vi "Extractor de bloobs.vi"() -> ()   [LabVIEW 2012]
doc: "Use this template to build a producer/consumer design pattern. Use this template when you need to execute a process, such as data analysis, when a data source, such as a triggered acquisition, produces data at an uneven rate and you need to execute the process when the data becomes available."
uses:
  <vilib>/vision/Image Controls.llb/IMAQ Image.ctl
  <vilib>/vision/NI_Vision_Development_Module.lvlib
panel:
  in  "Forma":i32=9
  in  "Tamaño":i32=50
  in  "Aguacate":bool
  out "Guardado":bool
  in  "Guardar":bool
  out "Image 2":T1(plugin-control)
  out "Cuadro":i32[](array[numeric])
  out "Image":T1(plugin-control)
  in  "Image\n  Path":path
  in  "stop":bool
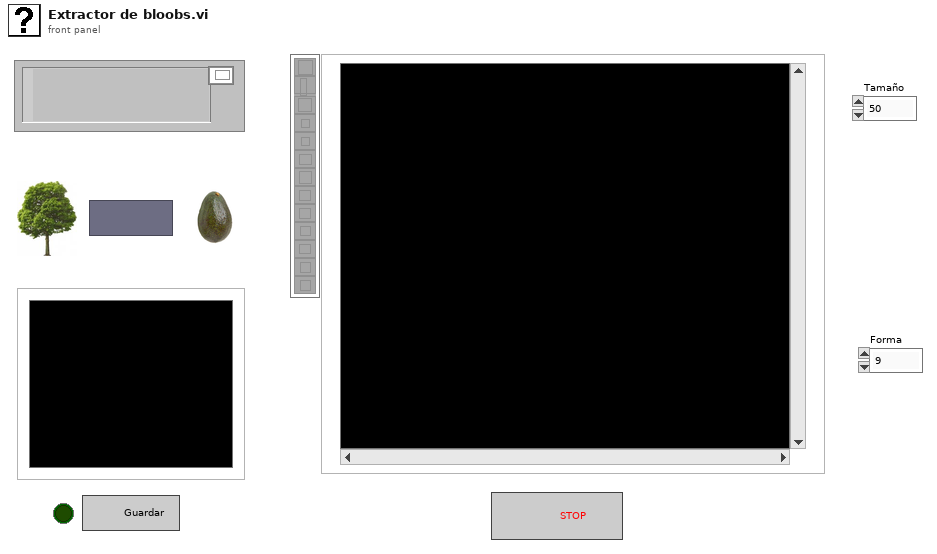
[diagram p1: front panel]
types:
  T1 = typedef "IMAQ Image.ctl" = refnum<image>
  T2 = cluster{"Global Rectangle":i32[], "Contours":cluster{"Contour Type":u32, "ROI Type":u32, "Points":i32[]}[]}
  T3 = cluster{"Contour Type":u32, "ROI Type":u32, "Points":i32[]}[]
  T4 = cluster{"Contour Type":u32, "ROI Type":u32, "Points":i32[]}
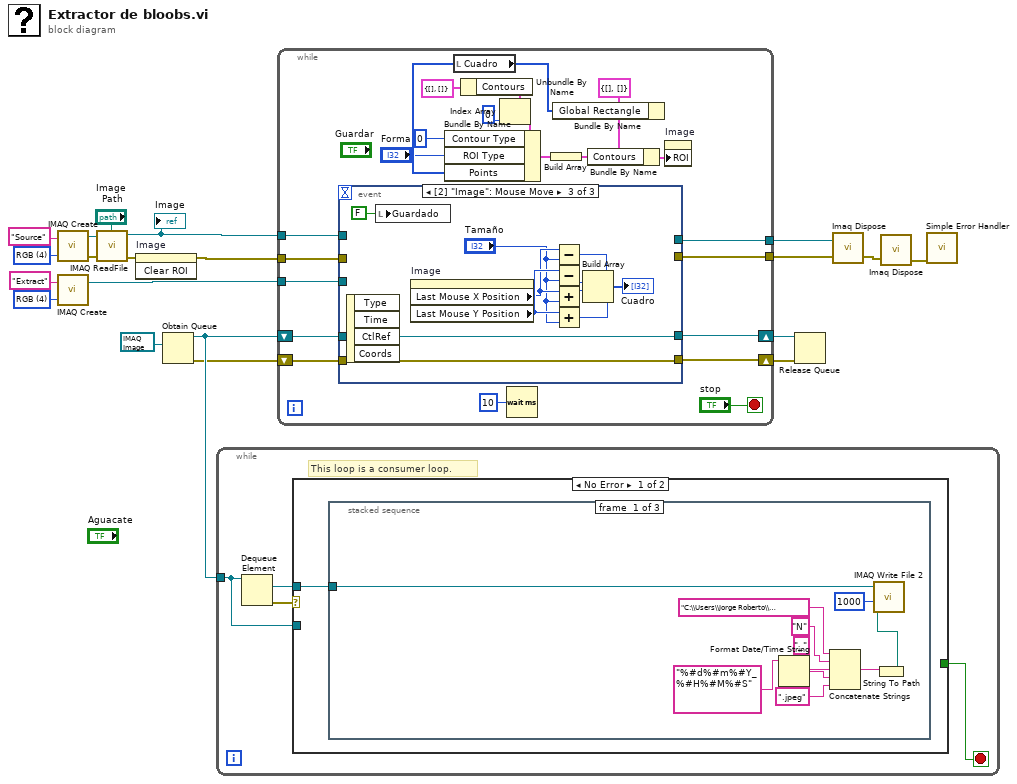
[diagram p0: block diagram]
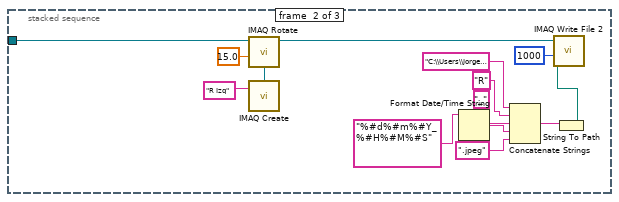
[diagram p2: hidden frame]
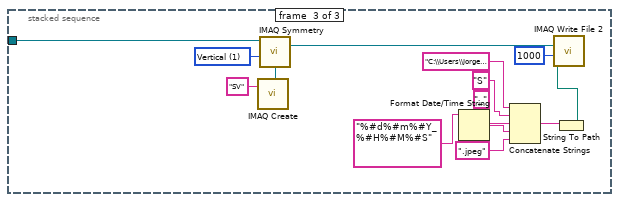
[diagram p3: hidden frame]
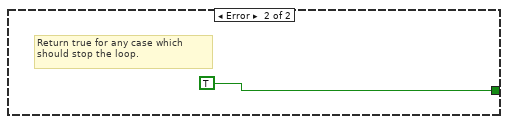
[diagram p4: hidden frame]
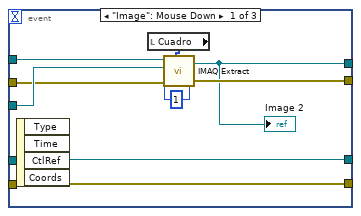
[diagram p5: hidden frame]
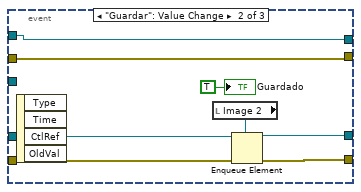
[diagram p6: hidden frame]
diagram:
  w16 = u32 4 items=["8 bits", "16 bits", "Float", "Complex", "RGB", "HSL"] ("Image Type")
  w15 = u32 4 items=["8 bits", "16 bits", "Float", "Complex", "RGB", "HSL"] ("Image Type")
  n1 = call "IMAQ Create"("Image Name"="Source", "Image Type"=w15) -> ("New Image"=w12:T1, "error out"=w11:errorcluster)  [unwired: 2 in, 1 out]
  n2 = call "IMAQ Create"("Image Name"="Extract", "Image Type"=w16) -> ("New Image"=w4:T1)  [unwired: 2 in, 2 out]
  n3 = call "IMAQ ReadFile"("File Path"="Image\n  Path", "error in (no error)"=w11, "Image"=w12) -> ("error out"=w9:errorcluster, "Image Out"=w3:T1)  [unwired: 2 in, 5 out]
  "Image" <- w3
  n4 = invoke on="Image" class="ImageControl" method="Clear ROI"(error in=w9) -> (error out=w5:errorcluster)  [unwired: 2 in, 2 out]
  n5 = Obtain Queue(element data type=T1 refnum ("Image")) -> (queue out=w20:refnum<queue>, error out=w19:errorcluster)  [unwired: 4 in, 1 out]
  n6 = while {
    tunnel: w20 -> [w21]
    stop <- w22 stop-if-true
    # "This loop is a consumer loop."
    n7 = Dequeue Element(queue=w21) -> (element=w23:T1, error out=w24:errorcluster)  [unwired: 2 in, 2 out]
    n8 = case shown="No Error" w24 {
      tunnel: w23 -> [w25 _]
      tunnel: [_ TRUE] -> w22
      tunnel: w21 -> [_ _]
      frame No Error {
        n9 = stacked-sequence {
          tunnel: w25 -> [w35 w49 w63]
          frame #0 {
            n10 = Format Date/Time String(time format string (%c)="%#d%#m%#Y_%#H%#M%#S") -> (date/time string=w34:string)  [unwired: 2 in]
            n11 = Concatenate Strings("C:\\Users\\Jorge Roberto\\Documents\\Aguacates\\Programa\\Blobs\\Normal\\", "N", "_", w34, ".jpeg") -> (w31:string)
            n12 = String To Path(string=w31) -> (path=w30:path)
            n13 = call-poly "IMAQ Write File 2"("Image Quality"=u32 1000, "File Path"=w30, "Image"=w35) -> ()  [unwired: 7 in, 2 out]
          }
          frame #1 {
            n14 = call "IMAQ Create"("Image Name"="R Izq") -> ("New Image"=w46:T1)  [unwired: 3 in, 2 out]
            n15 = call "IMAQ Rotate"("Angle (degrees)"=sgl 15.0, "Image Dst"=w46, "Image Src"=w49) -> ("Image Dst Out"=w36:T1)  [unwired: 7 in, 1 out]
            n16 = Format Date/Time String(time format string (%c)="%#d%#m%#Y_%#H%#M%#S") -> (date/time string=w45:string)  [unwired: 2 in]
            n17 = Concatenate Strings("C:\\Users\\Jorge Roberto\\Documents\\Aguacates\\Programa\\Blobs\\Simetrica\\", "R", "_", w45, ".jpeg") -> (w42:string)
            n18 = String To Path(string=w42) -> (path=w41:path)
            n19 = call-poly "IMAQ Write File 2"("Image Quality"=u32 1000, "File Path"=w41, "Image"=w36) -> ()  [unwired: 7 in, 2 out]
          }
          frame #2 {
            w62 = u32 1 items=["Horizontal", "Vertical", "Central", "1st Diagonal", "2nd Diagonal"] ("Type of Symmetry")
            n20 = call "IMAQ Create"("Image Name"="SV") -> ("New Image"=w51:T1)  [unwired: 3 in, 2 out]
            n21 = call "IMAQ Symmetry"("Type of Symmetry"=w62, "Image Dst"=w51, "Image Src"=w63) -> ("Image Dst Out"=w52:T1)  [unwired: 2 in, 1 out]
            n22 = Format Date/Time String(time format string (%c)="%#d%#m%#Y_%#H%#M%#S") -> (date/time string=w61:string)  [unwired: 2 in]
            n23 = Concatenate Strings("C:\\Users\\Jorge Roberto\\Documents\\Aguacates\\Programa\\Blobs\\Simetrica\\", "S", "_", w61, ".jpeg") -> (w58:string)
            n24 = String To Path(string=w58) -> (path=w57:path)
            n25 = call-poly "IMAQ Write File 2"("Image Quality"=u32 1000, "File Path"=w57, "Image"=w52) -> ()  [unwired: 7 in, 2 out]
          }
        }
      }
      frame Error {
        # "Return true for any case which should stop the loop."
      }
    }
  }
  n26 = while {
    shift-right: [w83] -> w17
    shift-left: w19 -> [w84]
    shift-right: [w85] -> w18
    shift-left: w20 -> [w86]
    tunnel: w5 -> [w79]
    tunnel: w4 -> [w80]
    tunnel: w3 -> [w81]
    tunnel: [w78] -> w2
    tunnel: [w77] -> w1
    stop <- "stop" stop-if-true
    n27 = event shown="[2] \"Image\": Mouse Move" {
      selector: _ -> [_ _ _]
      dyn-events: _ -> [_ _ _]
      timeout: _ -> [_ _ _]
      tunnel: w86 -> [w89 w101 w115]
      tunnel: [w89 w104 w115] -> w85
      tunnel: w84 -> [w88 w102 w114]
      tunnel: [w88 w103 w114] -> w83
      tunnel: w81 -> [w94 w99 _]
      tunnel: w80 -> [w93 _ _]
      tunnel: w79 -> [w92 w98 _]
      tunnel: [w90 w99 _] -> w78
      tunnel: [w91 w98 _] -> w77
      event "Image": Mouse Down {
        w95 = u32 1 ("Y Step")
        n28 = event-data() -> ()  [unwired: 1 in, 4 out]
        n29 = local read "Cuadro"() -> (w96:i32[])
        n30 = call "IMAQ Extract"("Y Step Size"=w95, "Optional Rectangle"=w96, "error in (no error)"=w92, "X Step Size"=w95, "Image Dst"=w93, "Image Src"=w94) -> ("error out"=w91:errorcluster, "Image Dst Out"=w90:T1)  [unwired: 4 out]
        "Image 2" <- w90
      }
      event "Guardar": Value Change {
        n31 = event-data() -> ()  [unwired: 1 in, 4 out]
        n32 = local read "Image 2"() -> (w100:T1)
        n33 = Enqueue Element(queue=w101, element=w100, error in (no error)=w102) -> (queue out=w104:refnum<queue>, error out=w103:errorcluster)  [unwired: 1 in, 1 out]
        "Guardado" <- TRUE ("Guardado")
      }
      event "Image": Mouse Move {
        n34 = event-data() -> ()  [unwired: 1 in, 4 out]
        n35 = local write "Guardado"(FALSE ("Guardado")) -> ()
        n36 = property on="Image" class="ImageControl"() -> ("Last Mouse X Position"=w107:i32, "Last Mouse Y Position"=w108:i32)  [unwired: 2 in, 2 out]
        n37 = Subtract(x=w107, y="Tamaño") -> (x-y=w110:i32)
        n38 = Subtract(x=w108, y="Tamaño") -> (x-y=w109:i32)
        n39 = Add(x=w107, y="Tamaño") -> (x+y=w112:i32)
        n40 = Add(x=w108, y="Tamaño") -> (x+y=w113:i32)
        n41 = Build Array(w110, w109, w112, w113) -> (→"Cuadro":i32[])
      }
    }
    n42 = local read "Cuadro"() -> (w70:i32[])
    n43 = Unbundle By Name(T2 {"Global Rectangle"=[], "Contours"=[]} ("ROI")) -> ("Contours"=w66:T3)
    n44 = Index Array(array=w66, index=0) -> (element=w68:T4)
    n45 = Bundle By Name(cluster=w68, "Contour Type"=0 ("index"), "ROI Type"="Forma", "Points"=w70) -> (w72:T4)
    n46 = Wait (ms)(milliseconds to wait=u32 10) -> ()  [unwired: 1 out]
    n47 = Build Array(w72) -> (w73:T3)
    n48 = Bundle By Name(cluster=T2 {"Global Rectangle"=[], "Contours"=[]} ("ROI"), "Global Rectangle"=w70) -> (w71:T2)
    n49 = Bundle By Name(cluster=w71, "Contours"=w73) -> (w76:T2)
    n50 = property on="Image" class="ImageControl"("ROI"=w76) -> ()  [unwired: 2 in, 2 out]
  }
  n51 = Release Queue(queue=w18, error in (no error)=w17) -> ()  [unwired: 1 in, 3 out]
  n52 = call "Imaq Dispose"("Image"=w2, "error in (no error)"=w1) -> ("error out"=w7:errorcluster)  [unwired: 1 in, 3 out]
  n53 = call "Imaq Dispose"("error in (no error)"=w7) -> ("error out"=w6:errorcluster)  [unwired: 2 in, 3 out]
  n54 = call <vilib>:"Simple Error Handler.vi"("error in (no error)"=w6) -> ()  [unwired: 1 in, 8 out]
